vi "FPGA Target Approach RetractionA2.vi"() -> ()   [LabVIEW 2012]
uses:
  <vilib>/rvi/FXPMathLib/basic elements/FxpIntAccumulator/subVIs/nifxpmath_IntAccumulator_SimConfig.ctl
  <vilib>/rvi/Emulation/niFpgaSctlEmulationGetInTimedLoop.vi
  <vilib>/rvi/Emulation/niFpgaSctlEmulationGlobalWrite.vi
  <vilib>/rvi/interface/RandomDataEmulation/nirviRandomDataFPGAFIFO.vi
  <vilib>/rvi/interface/RandomDataEmulation/niFpgaRandomDataHandleErrors.vi
  <vilib>/rvi/eio/common/nirviEmuTemplateMethod_errors.vi
  <vilib>/rvi/FXPMathLib/basic elements/FxpIntAccumulator/simVIs/DllFxpIntAccumulator_sub.vi
  <vilib>/rvi/DataTransferAndStorage/Container/XNode/niFpgaContainer.xnode
  <vilib>/rvi/interface/RandomDataEmulation/nirviRandomDataFpgaReadWriteTemplate.vi
  <vilib>/eio/EIONode/EIONode.xnode
  <vilib>/rvi/Analysis/measure/butterworth/XNode/niFpgaButterworthFilter.xnode
  <vilib>/rvi/FXPMathLib/basic elements/FxpIntAccumulator/XNode/nifxpmath_IntAccumulator.xnode
panel:
  out "Case 1":i16
  out "Case 3":i16
  out "Case 4":i16
  out "Case 2":i16
  out "Numeric 4":i32
  out "Numeric 3":i32
  out "Numeric 2":i32
  out "Numeric":i32
  in  "TF in Air":i32
  in  "Approach Minimum":i32
  in  "Approach Setpoint":i32
  in  "Fast Approach Offset":i32
  out "SummationfA":fxp<+/-,64,38>
  in  "Fine Approach Speed":fxp<+,64,38>
  out "SummationfR":fxp<+/-,64,38>
  in  "Fine Retraction Speed":fxp<+,64,38>
  out "SummationFA":fxp<+/-,64,38>
  out "Test Case Number Indicator":i16
  in  "Fast Approach Speed":fxp<+,64,38>
  in  "Manual":bool
  in  "Approach":bool
  out "SummationFR":fxp<+/-,64,38>
  in  "Data Acquisition Rate":i16
  out "Ticks":i16
  out "HV/10":i16
  out "Tuning Fork Signal":fxp<+/-,24,17>
  in  "Fast Retraction Speed":fxp<+,64,38>
  out "FPGA Output Voltage":fxp<+/-,64,32>
  out "Z Fine Indicator":fxp<+/-,40,30>
  out "Counter Indicator":fxp<+/-,64,32>
  in  "Z Fine Output":fxp<+/-,40,30>
  in  "Counter Output":i32
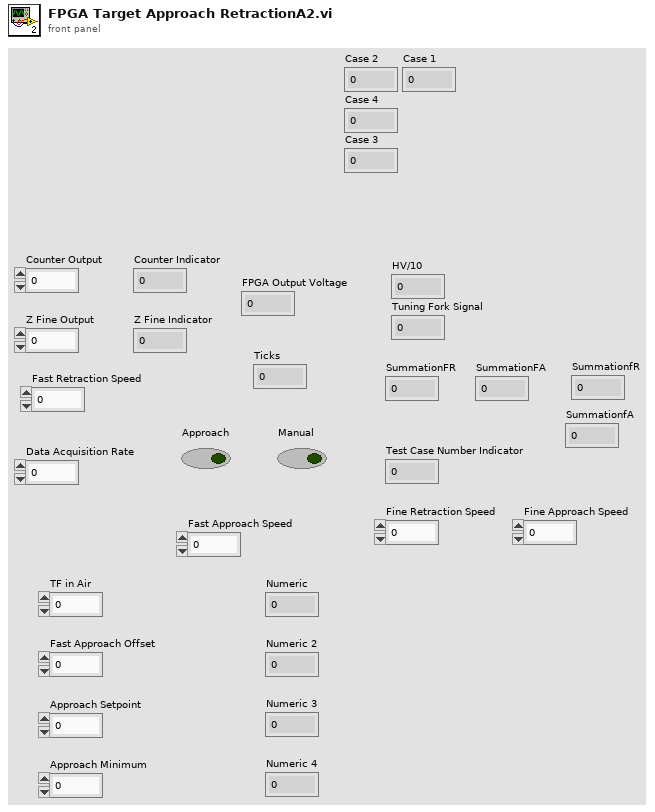
[diagram p1: front panel]
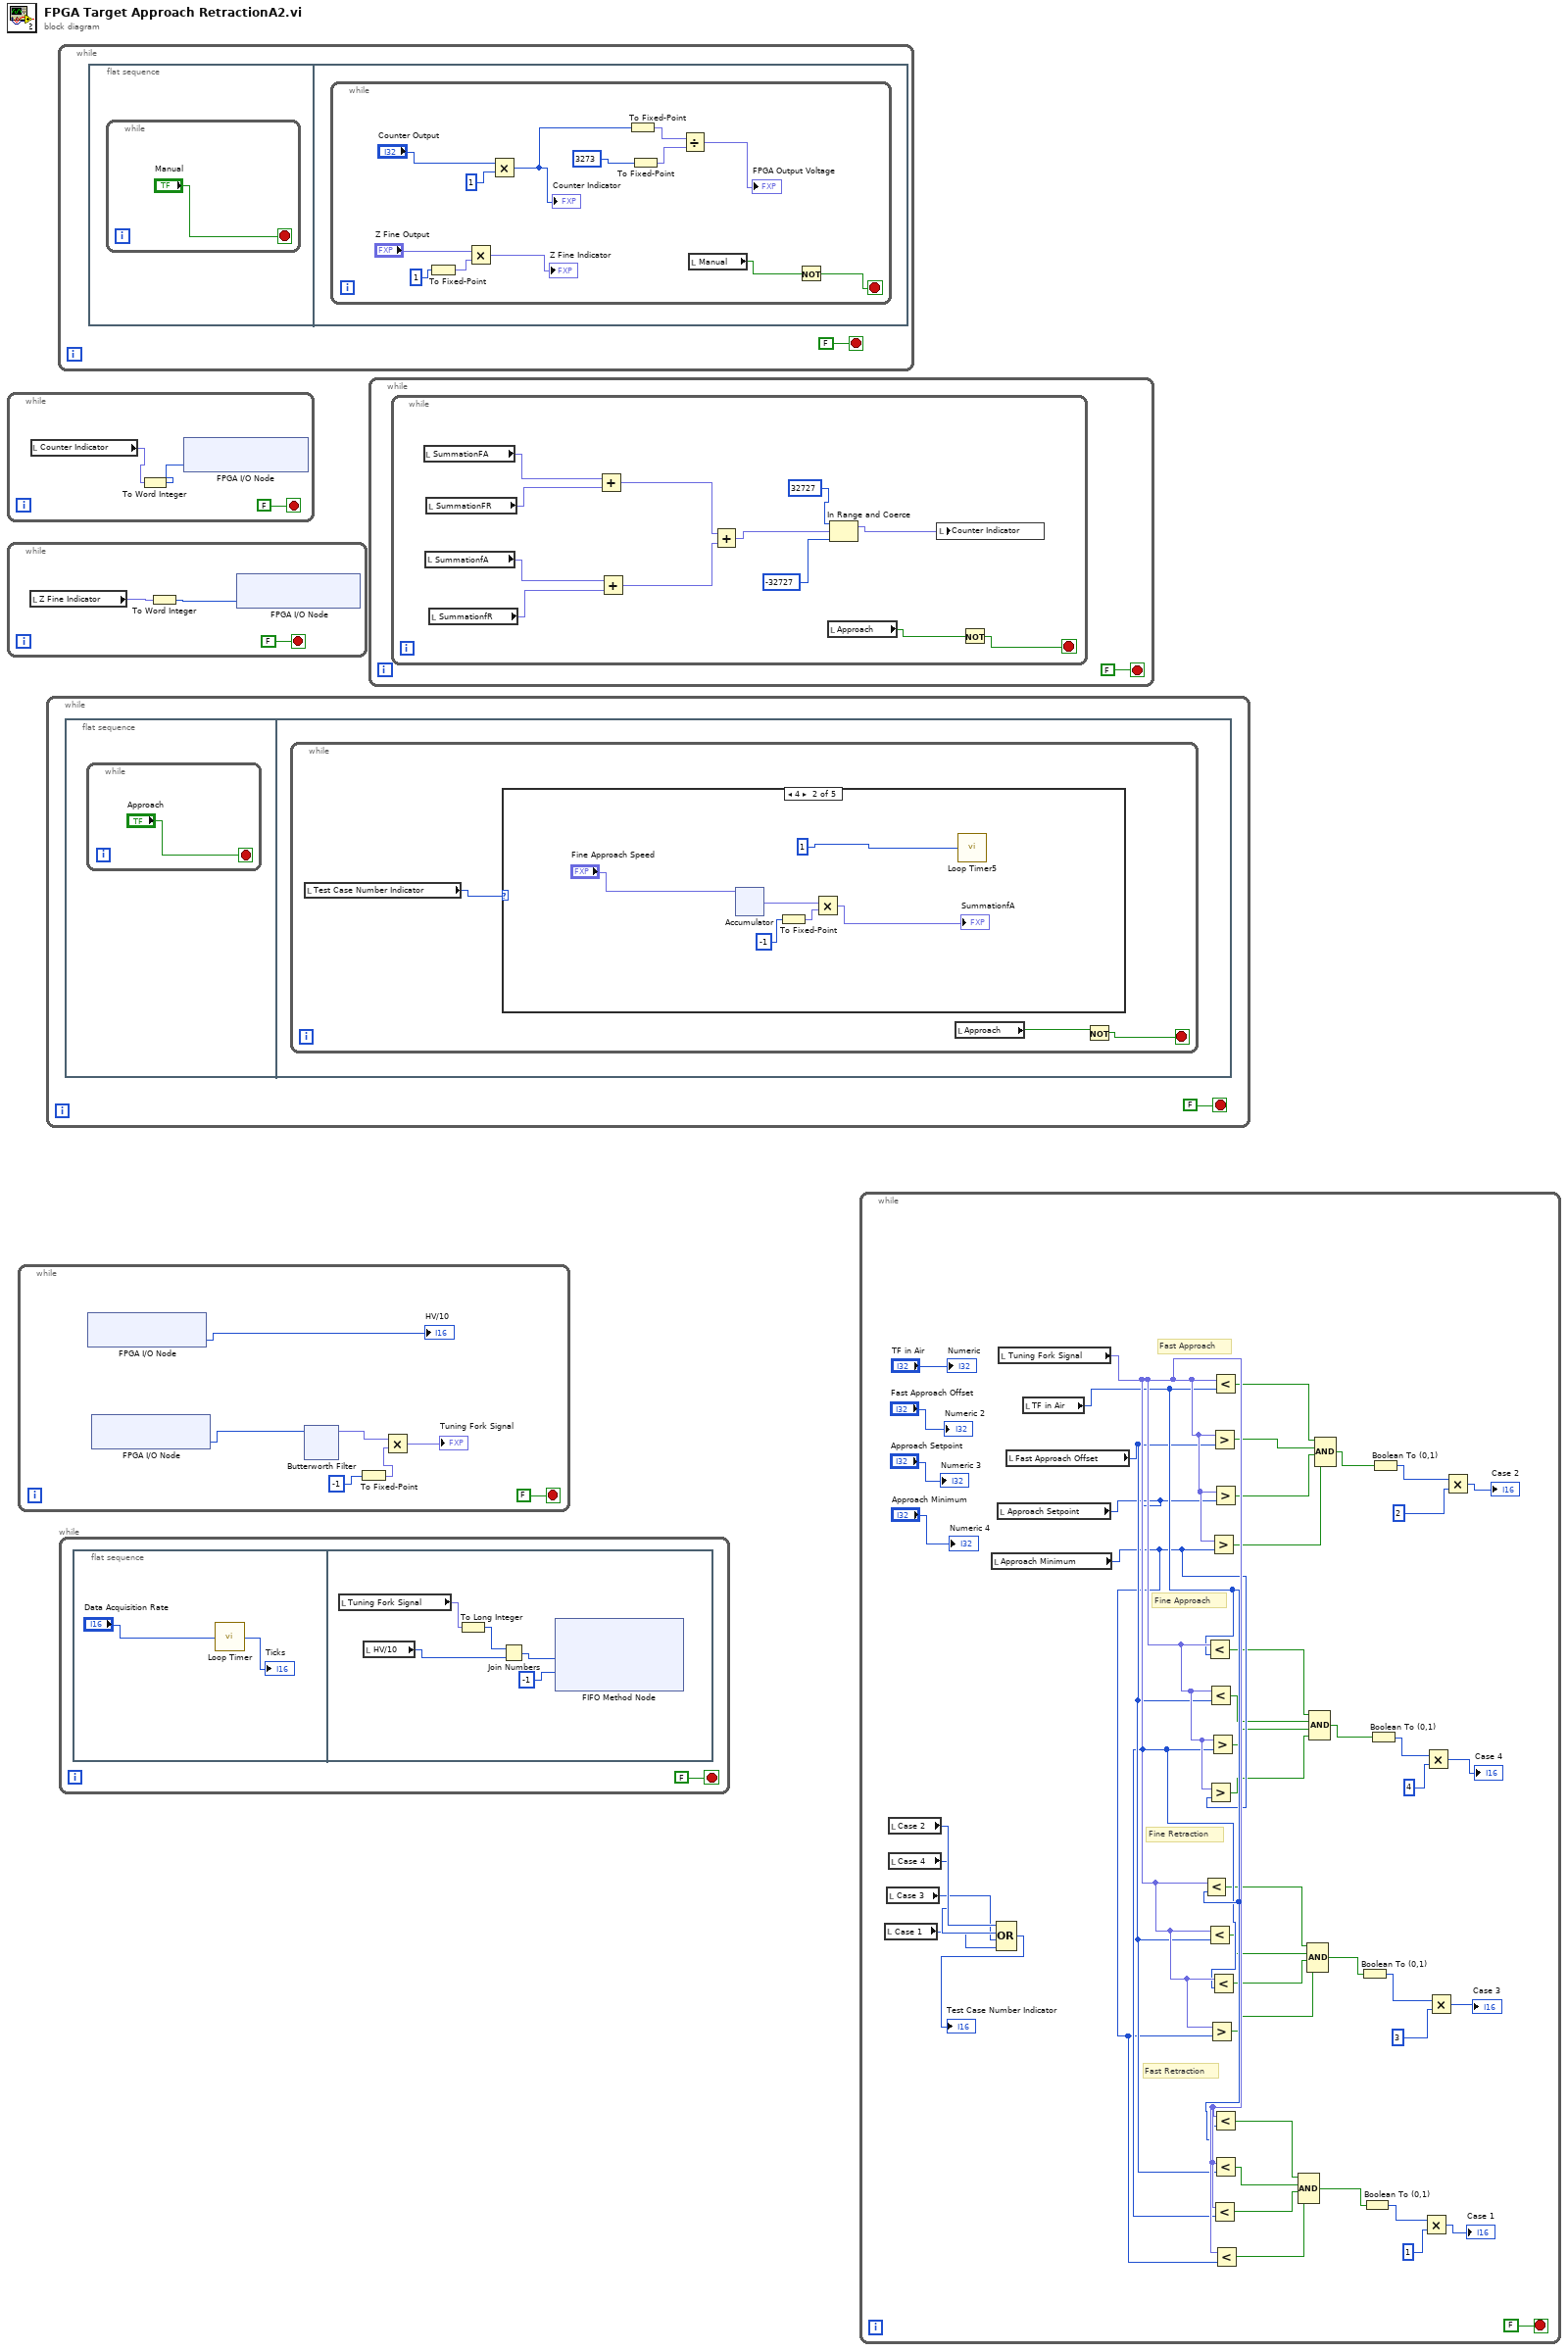
[diagram p0: block diagram]
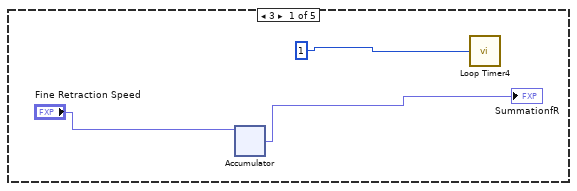
[diagram p2: hidden frame]
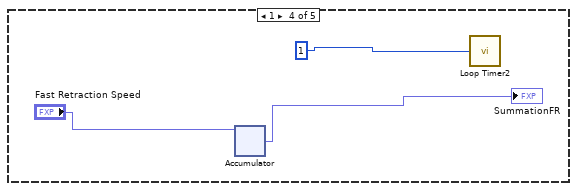
[diagram p4: hidden frame]
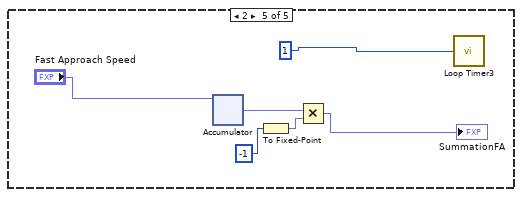
[diagram p5: hidden frame]
diagram:
  n1 = while {
    stop <- FALSE stop-if-true
    n2 = local read "Counter Indicator"() -> (w2:fxp<+/-,64,32>)
    n3 = To Word Integer(number=w2) -> (16bit integer=w1:i16)
    n4 = xnode "FPGA I/O Node"("Connector0/AO7"=w1) -> ()  [unwired: 1 in, 1 out]
  }
  n5 = while {
    stop <- FALSE stop-if-true
    n6 = local read "Z Fine Indicator"() -> (w5:fxp<+/-,40,30>)
    n7 = To Word Integer(number=w5) -> (16bit integer=w4:i16)
    n8 = xnode "FPGA I/O Node"("Connector0/AO2"=w4) -> ()  [unwired: 1 in, 1 out]
  }
  n9 = while {
    stop <- FALSE stop-if-true
    n10 = xnode "FPGA I/O Node"() -> ("Connector0/AI6"=→"HV/10":i16)  [unwired: 1 in, 1 out]
    n11 = xnode "FPGA I/O Node"() -> ("Connector0/AI7"=w12:i16)  [unwired: 1 in, 1 out]
    n12 = xnode "Butterworth Filter"("input data"=w12) -> ("output data"=w8:fxp<+/-,20,20>)  [unwired: 2 in]
    n13 = To Fixed-Point(number=i16 -1) -> (fixed-point=w9:fxp<+/-,16,16>)  [unwired: 1 in]
    n14 = Multiply(x=w8, y=w9) -> (x*y=→"Tuning Fork Signal":fxp<+/-,36,36>)
  }
  n15 = while {
    stop <- FALSE stop-if-true
    n16 = flat-sequence {
      frame #0 {
        n17 = while {
          stop <- "Approach" stop-if-true
        }
      }
      frame #1 {
        n18 = while {
          stop <- w24 stop-if-true
          n19 = local read "Test Case Number Indicator"() -> (w23:i16)
          n20 = case shown="4" w23 {
            frame 3 {
              n21 = xnode "Accumulator"("x"="Fine Retraction Speed") -> ("s"=→"SummationfR":fxp<+,64,38>)  [unwired: 4 in, 1 out]
              n22 = call "Loop Timer4"("Count(uSec)"=i16 1) -> ()  [unwired: 1 out]
            }
            frame 4 {
              n23 = xnode "Accumulator"("x"="Fine Approach Speed") -> ("s"=w60:fxp<+,64,38>)  [unwired: 4 in, 1 out]
              n24 = To Fixed-Point(number=i16 -1) -> (fixed-point=w58:fxp<+/-,16,16>)  [unwired: 1 in]
              n25 = Multiply(x=w60, y=w58) -> (x*y=→"SummationfA":fxp<+/-,64,54>)
              n26 = call "Loop Timer5"("Count(uSec)"=i16 1) -> ()  [unwired: 1 out]
            }
            frame 5, Default {
            }
            frame 1 {
              n27 = xnode "Accumulator"("x"="Fast Retraction Speed") -> ("s"=→"SummationFR":fxp<+,64,38>)  [unwired: 4 in, 1 out]
              n28 = call "Loop Timer2"("Count(uSec)"=i16 1) -> ()  [unwired: 1 out]
            }
            frame 2 {
              n29 = xnode "Accumulator"("x"="Fast Approach Speed") -> ("s"=w120:fxp<+,64,38>)  [unwired: 4 in, 1 out]
              n30 = To Fixed-Point(number=i16 -1) -> (fixed-point=w122:fxp<+/-,16,16>)  [unwired: 1 in]
              n31 = Multiply(x=w120, y=w122) -> (x*y=→"SummationFA":fxp<+/-,64,54>)
              n32 = call "Loop Timer3"("Count(uSec)"=i16 1) -> ()  [unwired: 1 out]
            }
          }
          n33 = local read "Approach"() -> (w25:bool)
          n34 = Not(x=w25) -> (.not. x?=w24:bool)
        }
      }
    }
  }
  n35 = while {
    stop <- FALSE stop-if-true
    n36 = flat-sequence {
      frame #0 {
        n37 = while {
          stop <- "Manual" stop-if-true
        }
      }
      frame #1 {
        n38 = while {
          stop <- w154 stop-if-true
          n39 = To Fixed-Point(number=1) -> (fixed-point=w162:fxp<+/-,32,32>)  [unwired: 1 in]
          n40 = Multiply(x="Z Fine Output", y=w162) -> (x*y=→"Z Fine Indicator":fxp<+/-,64,62>)
          n41 = Multiply(x="Counter Output", y=1) -> (x*y=w160:i32)
          "Counter Indicator" <- w160
          n42 = To Fixed-Point(number=w160) -> (fixed-point=w159:fxp<+/-,32,32>)  [unwired: 1 in]
          n43 = To Fixed-Point(number=3273) -> (fixed-point=w158:fxp<+/-,32,32>)  [unwired: 1 in]
          n44 = Divide(x=w159, y=w158) -> (x/y=→"FPGA Output Voltage":fxp<+/-,64,33>)
          n45 = local read "Manual"() -> (w155:bool)
          n46 = Not(x=w155) -> (.not. x?=w154:bool)
        }
      }
    }
  }
  n47 = while {
    stop <- FALSE stop-if-true
    n48 = flat-sequence {
      frame #0 {
        n49 = call "Loop Timer"("Count(uSec)"="Data Acquisition Rate") -> ("Tick Count(uSec)"=→"Ticks":u32)
      }
      frame #1 {
        n50 = local read "Tuning Fork Signal"() -> (w174:fxp<+/-,24,17>)
        n51 = local read "HV/10"() -> (w173:i16)
        n52 = To Long Integer(number=w174) -> (32bit integer=w172:i32)
        n53 = Join Numbers(hi=w172, lo=w173) -> ((hi.lo)=w171:u64)
        n54 = xnode ("FIFO Method Node")("Element"=w171, "Timeout"=i16 -1) -> ()  [unwired: 1 in, 2 out]
      }
    }
  }
  n55 = while {
    stop <- FALSE stop-if-true
    n56 = while {
      stop <- w176 stop-if-true
      n57 = local read "SummationFA"() -> (w187:fxp<+/-,64,38>)
      n58 = local read "SummationfA"() -> (w185:fxp<+/-,64,38>)
      n59 = local read "SummationFR"() -> (w186:fxp<+/-,64,38>)
      n60 = local read "SummationfR"() -> (w184:fxp<+/-,64,38>)
      n61 = Add(x=w187, y=w186) -> (x+y=w182:fxp<+/-,64,39>)
      n62 = Add(x=w185, y=w184) -> (x+y=w183:fxp<+/-,64,39>)
      n63 = Add(x=w182, y=w183) -> (x+y=w181:fxp<+/-,64,40>)
      n64 = local read "Approach"() -> (w177:bool)
      n65 = In Range and Coerce(upper limit=i16 32727, x=w181, lower limit=i16 -32727) -> (coerced(x)=w178:fxp<+/-,64,40>)  [unwired: 1 out]
      n66 = local write "Counter Indicator"(w178) -> ()
      n67 = Not(x=w177) -> (.not. x?=w176:bool)
    }
  }
  n68 = while {
    stop <- FALSE stop-if-true
    # "Fast Retraction"
    # "Fine Retraction"
    # "Fine Approach"
    # "Fast Approach"
    n69 = local read "Case 1"() -> (w188:i16)
    n70 = local read "Case 3"() -> (w189:i16)
    n71 = local read "Case 2"() -> (w191:i16)
    n72 = local read "Case 4"() -> (w190:i16)
    n73 = local read "Approach Minimum"() -> (w225:i32)
    n74 = Compound Arithmetic op=OR(w191, w190, w189, w188) -> (→"Test Case Number Indicator":i16)
    n75 = local read "Approach Setpoint"() -> (w226:i32)
    n76 = local read "Tuning Fork Signal"() -> (w229:fxp<+/-,24,17>)
    n77 = local read "Fast Approach Offset"() -> (w227:i32)
    n78 = local read "TF in Air"() -> (w228:i32)
    n79 = Less?(x=w229, y=w228) -> (x < y?=w214:bool)
    n80 = Less?(x=w229, y=w228) -> (x < y?=w219:bool)
    n81 = Less?(x=w229, y=w227) -> (x < y?=w213:bool)
    n82 = Less?(x=w229, y=w227) -> (x < y?=w218:bool)
    n83 = Greater?(x=w229, y=w225) -> (0:w216:bool)
    n84 = Greater?(x=w229, y=w225) -> (0:w211:bool)
    n85 = Greater?(x=w229, y=w226) -> (0:w217:bool)
    n86 = Greater?(x=w229, y=w225) -> (0:w221:bool)
    n87 = Less?(x=w229, y=w226) -> (x < y?=w212:bool)
    n88 = Greater?(x=w229, y=w227) -> (0:w223:bool)
    n89 = Less?(x=w229, y=w226) -> (x < y?=w207:bool)
    n90 = Less?(x=w229, y=w228) -> (x < y?=w224:bool)
    n91 = Greater?(x=w229, y=w226) -> (0:w222:bool)
    n92 = Less?(x=w229, y=w228) -> (x < y?=w209:bool)
    n93 = Less?(x=w229, y=w227) -> (x < y?=w208:bool)
    n94 = Less?(x=w229, y=w225) -> (x < y?=w206:bool)
    n95 = Compound Arithmetic op=AND(w209, w208, w207, w206) -> (w205:bool)
    n96 = Compound Arithmetic op=AND(w214, w213, w212, w211) -> (w210:bool)
    n97 = Compound Arithmetic op=AND(w219, w218, w217, w216) -> (w215:bool)
    n98 = Compound Arithmetic op=AND(w224, w223, w222, w221) -> (w220:bool)
    n99 = Boolean To (0,1)(Boolean=w210) -> (0, 1=w202:i16)
    n100 = Boolean To (0,1)(Boolean=w205) -> (0, 1=w201:i16)
    n101 = Boolean To (0,1)(Boolean=w215) -> (0, 1=w203:i16)
    n102 = Boolean To (0,1)(Boolean=w220) -> (0, 1=w204:i16)
    n103 = Multiply(x=w201, y=i16 1) -> (x*y=→"Case 1":i16)
    n104 = Multiply(x=w203, y=i16 4) -> (x*y=→"Case 4":i16)
    n105 = Multiply(x=w202, y=i16 3) -> (x*y=→"Case 3":i16)
    n106 = Multiply(x=w204, y=i16 2) -> (x*y=→"Case 2":i16)
    "Numeric" <- "TF in Air"
    "Numeric 2" <- "Fast Approach Offset"
    "Numeric 3" <- "Approach Setpoint"
    "Numeric 4" <- "Approach Minimum"
  }
